vi "Get Last Response Code.vi"(8 "error in (no error)":errorcluster, 11 "Response header":string) -> (0 "error out":errorcluster, 3 "Response code (last)":string)   [LabVIEW 2015, in "NI_AWS_Core.lvclass"]
doc: "Parses out the last HTTP result code (like 200, 404, 307...) as a string from a HTTP Response Header."
uses:
  NI_AWS_Core.lvclass
  <vilib>/regexp/Match Regular Expression.xnode
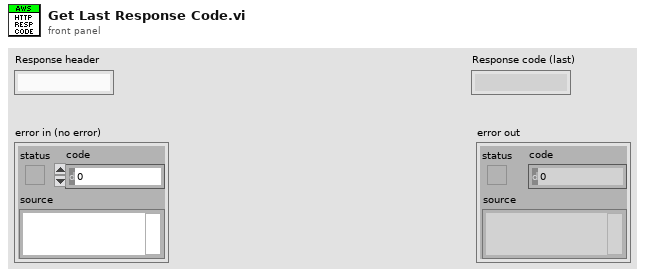
[diagram p1: front panel]
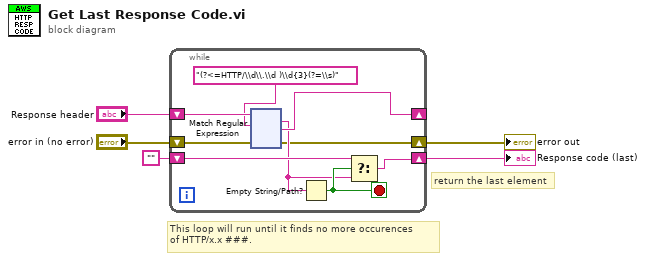
[diagram p0: block diagram]
diagram:
  # "return the last element"
  # "This loop will run until it finds no more occurences\nof HTTP/x.x ###."
  n1 = while {
    shift-right: [w12] -> _
    shift-left: "Response header" -> [w13]
    shift-right: [w9] -> w1
    shift-left: "" -> [w10]
    shift-right: [w6] -> w2
    shift-left: "error in (no error)" -> [w14]
    stop <- w11 stop-if-true
    n2 = xnode "Match Regular Expression"("input string"=w13, "regular expression"="(?<=HTTP/\\d\\.\\d )\\d{3}(?=\\s)", "error in"=w14) -> ("whole match"=w8:string, "after match"=w12:string, "error out"=w6:errorcluster)  [unwired: 3 in, 2 out]
    n3 = Empty String/Path?(string/path=w8) -> (empty?=w11:bool)
    n4 = Select(t=w10, s=w11, f=w8) -> (s? t:f=w9:string)
  }
  "Response code (last)" <- w1
  "error out" <- w2
